vi "RecursiveDirectoryStructureGenerator (SubVI).vi"(8 "error in (no error)":errorcluster, 10 "Folder index":i32, 11 "Host directory":path) -> (0 "error out":errorcluster, 3 "Nth subfolder in host directory":path)   [LabVIEW 2016]
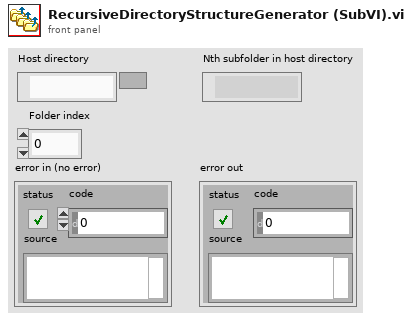
[diagram p1: front panel]
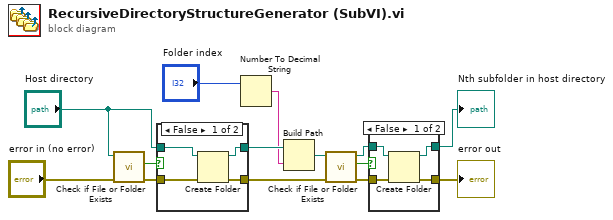
[diagram p0: block diagram]
diagram:
  n1 = call <vilib>:"Check if File or Folder Exists.vi"("error in (no error)"="error in (no error)", "path"="Host directory") -> ("error out"=w3:errorcluster, "file or folder exists?"=w1:bool)  [unwired: 7 in, 1 out]
  n2 = case shown="False" w1 {
    tunnel: "Host directory" -> [w18 w20]
    tunnel: [w17 w20] -> w10
    tunnel: w3 -> [w16 w19]
    tunnel: [w15 w19] -> w12
    frame False {
      n3 = Create Folder(path (use dialog)=w18, error in=w16) -> (created path=w17:path, error out=w15:errorcluster)  [unwired: 1 in, 1 out]
    }
    frame True {
    }
  }
  n4 = Number To Decimal String(number="Folder index") -> (decimal integer string=w9:string)  [unwired: 1 in]
  n5 = Build Path(base path=w10, name or relative path=w9) -> (appended path=w5:path)
  n6 = call <vilib>:"Check if File or Folder Exists.vi"("error in (no error)"=w12, "path"=w5) -> ("error out"=w6:errorcluster, "file or folder exists?"=w8:bool, "dup path"=w7:path)  [unwired: 7 in]
  n7 = case shown="False" w8 {
    tunnel: [w24 w25] -> w13
    tunnel: [w23 w26] -> w11
    tunnel: w7 -> [w22 w26]
    tunnel: w6 -> [w21 w25]
    frame False {
      n8 = Create Folder(path (use dialog)=w22, error in=w21) -> (created path=w23:path, error out=w24:errorcluster)  [unwired: 1 in, 1 out]
    }
    frame True {
    }
  }
  "error out" <- w13
  "Nth subfolder in host directory" <- w11
